vi "AtSpectrograph_logEvent_rejectedCommand.vi"(8 "error in (no error)":errorcluster, 11 "logevent_rejectedCommand_Ctl":T1) -> (0 "error out":errorcluster, 2 "function return":i32, 3 "logevent_rejectedCommand_Ctl out":T1)   [LabVIEW 2016, in "SALLV_AtSpectrograph.lvlib"]
doc: "int AtSpectrograph_shm_logEvent_rejectedCommandLV(AtSpectrograph_logevent_rejectedCommandLV *logevent_rejectedCommand_Ctl );"
uses:
  SALLV_AtSpectrograph.lvlib
  DataTypes/logevent_rejectedCommand.ctl
  SALLV_AtSpectrograph.so
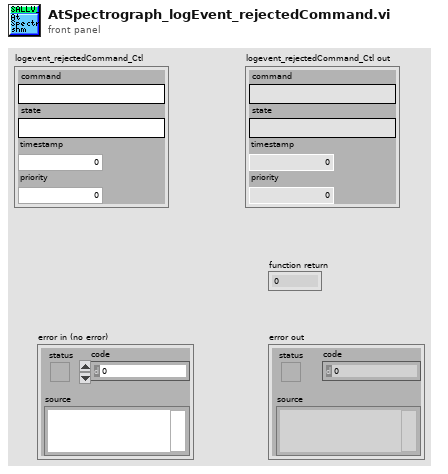
[diagram p1: front panel]
types:
  T1 = typedef "SALLV_AtSpectrograph.lvlib/logevent_rejectedCommand.ctl" = cluster{"command":string, "state":string, "timestamp":dbl, "priority":i32}
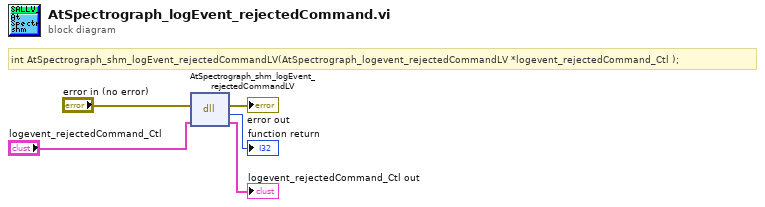
[diagram p0: block diagram]
diagram:
  # "int AtSpectrograph_shm_logEvent_rejectedCommandLV(AtSpectrograph_logevent_rejectedCommandLV *logevent_rejectedCommand_Ctl );"
  n1 = dll-call lib="home/harini/tcs/temp/SALLV_AtSpectrograph/SALLV_AtSpectrograph.*" fn="AtSpectrograph_shm_logEvent_rejectedCommandLV"(error in="error in (no error)", "logevent_rejectedCommand_Ctl"="logevent_rejectedCommand_Ctl") -> (error out=→"error out":errorcluster, →"function return":i32, "logevent_rejectedCommand_Ctl"=→"logevent_rejectedCommand_Ctl out":T1)  [unwired: 2 in, 1 out]
